vi "notM&s.vi"() -> ()   [LabVIEW 2022 SP3]
uses:
  12.ctl
panel:
  in  "slave 2":bool
  in  "slave 1":bool
  in  "stop":bool
  in  "input":i32
  out "slave 2":i32
  out "slave1":i32
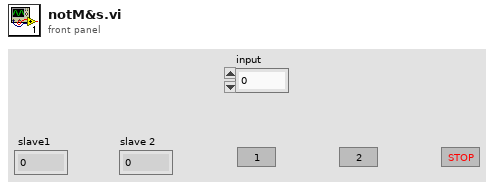
[diagram p1: front panel]
types:
  T1 = typedef "12.ctl" = enum16{"Poll", "Init", "Slave1", "Slave2", "Stop", "Error", "Exit"}
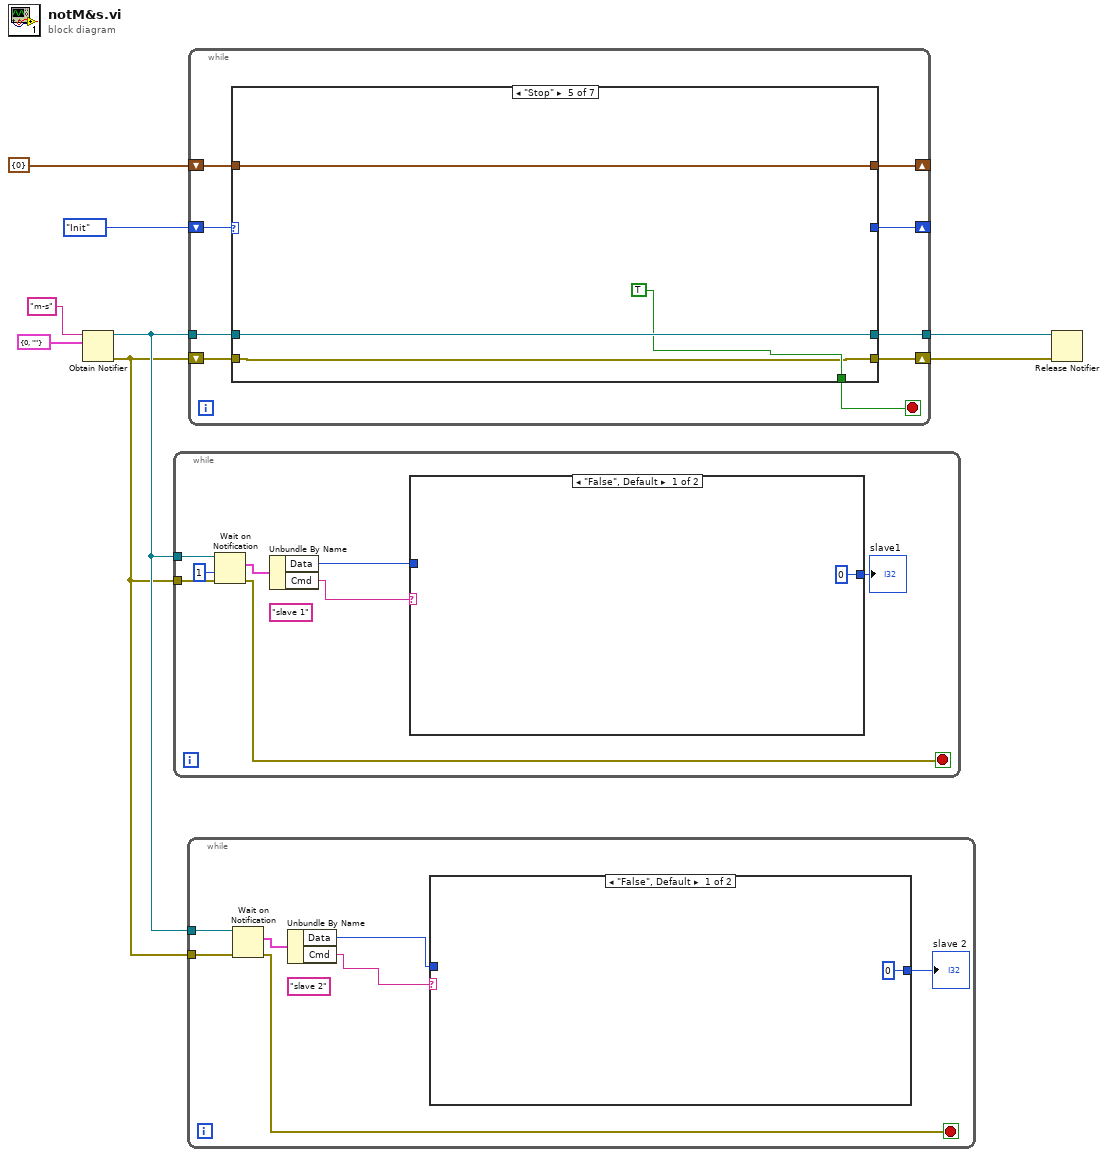
[diagram p0: block diagram]
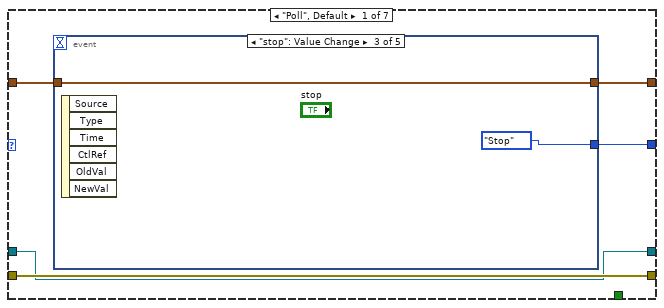
[diagram p4: hidden frame]
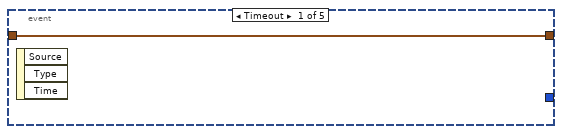
[diagram p5: hidden frame]
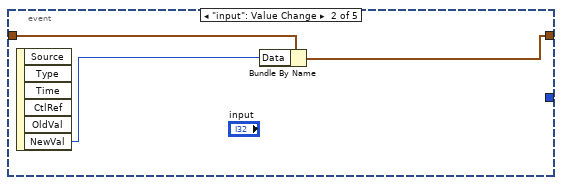
[diagram p6: hidden frame]
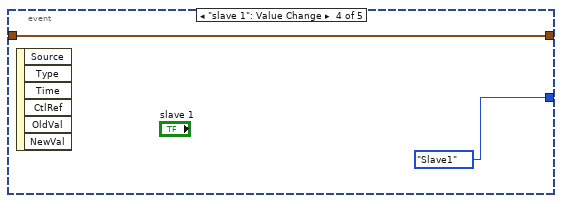
[diagram p7: hidden frame]
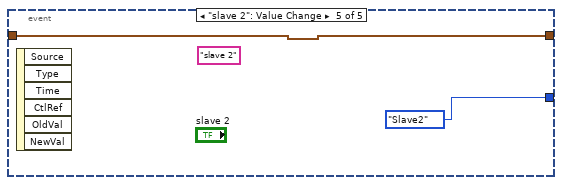
[diagram p8: hidden frame]
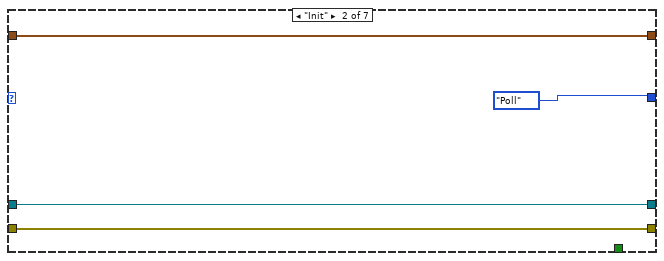
[diagram p9: hidden frame]
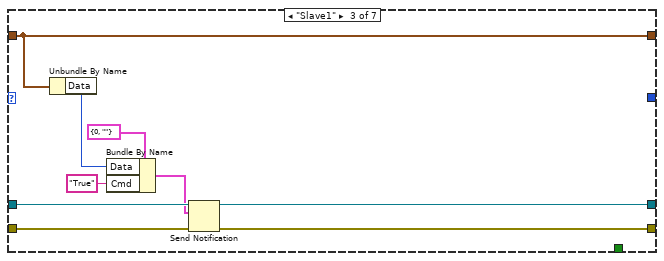
[diagram p10: hidden frame]
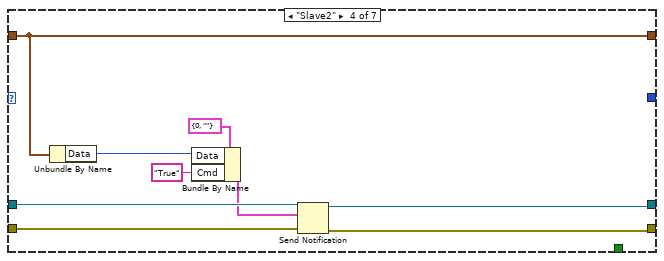
[diagram p11: hidden frame]
diagram:
  n1 = Obtain Notifier(name (unnamed)="m-s", notification data type=cluster{"Data":i32, "Cmd":string} {"Data"=0, "Cmd"=""}) -> (notifier out=w3:refnum<notifier>, error out=w2:errorcluster)  [unwired: 2 in, 1 out]
  n2 = while {
    tunnel: w3 -> [w16]
    tunnel: w2 -> [w15]
    stop <- w14 stop-if-true
    (unwired) "slave 1" ("y")
    n3 = Wait on Notification(notifier=w16, timeout in ms (-1)=1, error in (no error)=w15) -> (notification=w13:cluster{"Data":i32, "Cmd":string}, error out=w14:errorcluster)  [unwired: 1 in, 2 out]
    n4 = Unbundle By Name(w13) -> ("Data"=w11:i32, "Cmd"=w9:string)
    n5 = case shown="\"False\", Default" w9 {
      tunnel: [0 ("Data") w18] -> w12
      tunnel: w11 -> [_ w18]
      frame "False", Default {
      }
      frame "True" {
      }
    }
    "slave1" <- w12
  }
  n6 = while {
    tunnel: w3 -> [w25]
    tunnel: w2 -> [w24]
    stop <- w23 stop-if-true
    (unwired) "slave 2" ("y")
    n7 = Wait on Notification(notifier=w25, error in (no error)=w24) -> (notification=w22:cluster{"Data":i32, "Cmd":string}, error out=w23:errorcluster)  [unwired: 2 in, 2 out]
    n8 = Unbundle By Name(w22) -> ("Data"=w19:i32, "Cmd"=w21:string)
    n9 = case shown="\"False\", Default" w21 {
      tunnel: w19 -> [_ w27]
      tunnel: [0 ("Data") w27] -> w20
      frame "False", Default {
      }
      frame "True" {
      }
    }
    "slave 2" <- w20
  }
  n10 = while {
    shift-right: [w35] -> _
    shift-left: 12."Init" -> [w36]
    shift-right: [w34] -> _
    shift-left: cluster{"Data":i32} {"Data"=0} -> [w33]
    shift-right: [w30] -> w7
    shift-left: w2 -> [w31]
    tunnel: w3 -> [w29]
    tunnel: [w28] -> w6
    stop <- w32 stop-if-true
    n11 = case shown="\"Stop\"" w36 {
      tunnel: [w41 12."Poll" _ _ _ _ _] -> w35
      tunnel: [w40 w55 w58 w67 w77 w78 w83] -> w34
      tunnel: w33 -> [w39 w55 w58 w67 w77 w78 w83]
      tunnel: [_ _ _ _ TRUE _ _] -> w32
      tunnel: w31 -> [w38 w53 w64 w73 w74 w80 w82]
      tunnel: [w38 w53 w63 w72 w74 w80 w82] -> w30
      tunnel: w29 -> [w37 w52 w62 w71 w76 w79 w81]
      tunnel: [w37 w52 w61 w70 w76 w79 w81] -> w28
      frame "Poll", Default {
        n12 = event shown="[2] \"stop\": Value Change" {
          selector: _ -> [_ _ _ _ _]
          dyn-events: _ -> [_ _ _ _ _]
          timeout: _ -> [_ _ _ _ _]
          tunnel: [_ _ 12."Stop" 12."Slave1" 12."Slave2"] -> w41
          tunnel: [w42 w43 w46 w48 w50] -> w40
          tunnel: w39 -> [w42 w45 w46 w48 w50]
          event Timeout {
            n13 = event-data() -> ()  [unwired: 1 in, 3 out]
          }
          event "input": Value Change {
            n14 = event-data() -> ("NewVal"=w44:i32)  [unwired: 1 in, 5 out]
            n15 = Bundle By Name(cluster=w45, "Data"=w44) -> (w43:cluster{"Data":i32})
          }
          event "stop": Value Change {
            n16 = event-data() -> ()  [unwired: 1 in, 6 out]
          }
          event "slave 1": Value Change {
            n17 = event-data() -> ()  [unwired: 1 in, 6 out]
          }
          event "slave 2": Value Change {
            (unwired) "slave 2" ("Cmd")
            n18 = event-data() -> ()  [unwired: 1 in, 6 out]
          }
        }
      }
      frame "Init" {
      }
      frame "Slave1" {
        n19 = Unbundle By Name(w58) -> ("Data"=w57:i32)
        n20 = Bundle By Name(cluster=cluster{"Data":i32, "Cmd":string} {"Data"=0, "Cmd"=""}, "Data"=w57, "Cmd"="True") -> (w59:cluster{"Data":i32, "Cmd":string})
        n21 = Send Notification(notification=w59, notifier=w62, error in (no error)=w64) -> (notifier out=w61:refnum<notifier>, error out=w63:errorcluster)
      }
      frame "Slave2" {
        n22 = Unbundle By Name(w67) -> ("Data"=w66:i32)
        n23 = Bundle By Name(cluster=cluster{"Data":i32, "Cmd":string} {"Data"=0, "Cmd"=""} ("notification"), "Data"=w66, "Cmd"="True") -> (w68:cluster{"Data":i32, "Cmd":string})
        n24 = Send Notification(notification=w68, notifier=w71, error in (no error)=w73) -> (notifier out=w70:refnum<notifier>, error out=w72:errorcluster)
      }
      frame "Stop" {
      }
      frame "Error" {
      }
      frame "Exit" {
      }
    }
  }
  n25 = Release Notifier(notifier=w6, error in (no error)=w7) -> ()  [unwired: 1 in, 3 out]
